vi "DWE Get Time.vi"(9 "Date":string, 10 "# of rows":i32, 11 "Data row":string[][](array[string])) -> (3 "Time array":timestamp[](array[timestamp]))   [LabVIEW 2014]
doc: "Determine and record date of logged data (Laundry.NET does not provide date)."
panel:
  out "Array":bool[](array[boolean])
  out "Numeric":i32
  out "hour":string
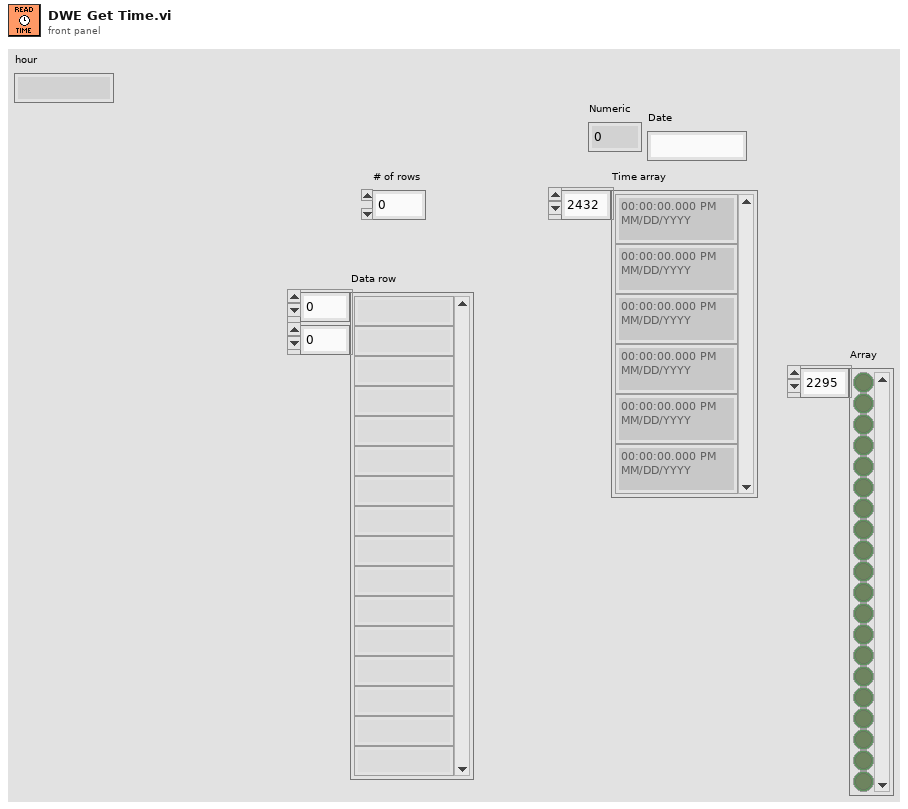
[diagram p1: front panel]
types:
  T1 = typedef "LVDateTimeRec.ctl" = cluster{"fractional second":dbl, "second":i32, "minute":i32, "hour":i32, "day of month":i32, "month":i32, "year":i32, "day of week":i32, "day of year":i32, "DST":i32}
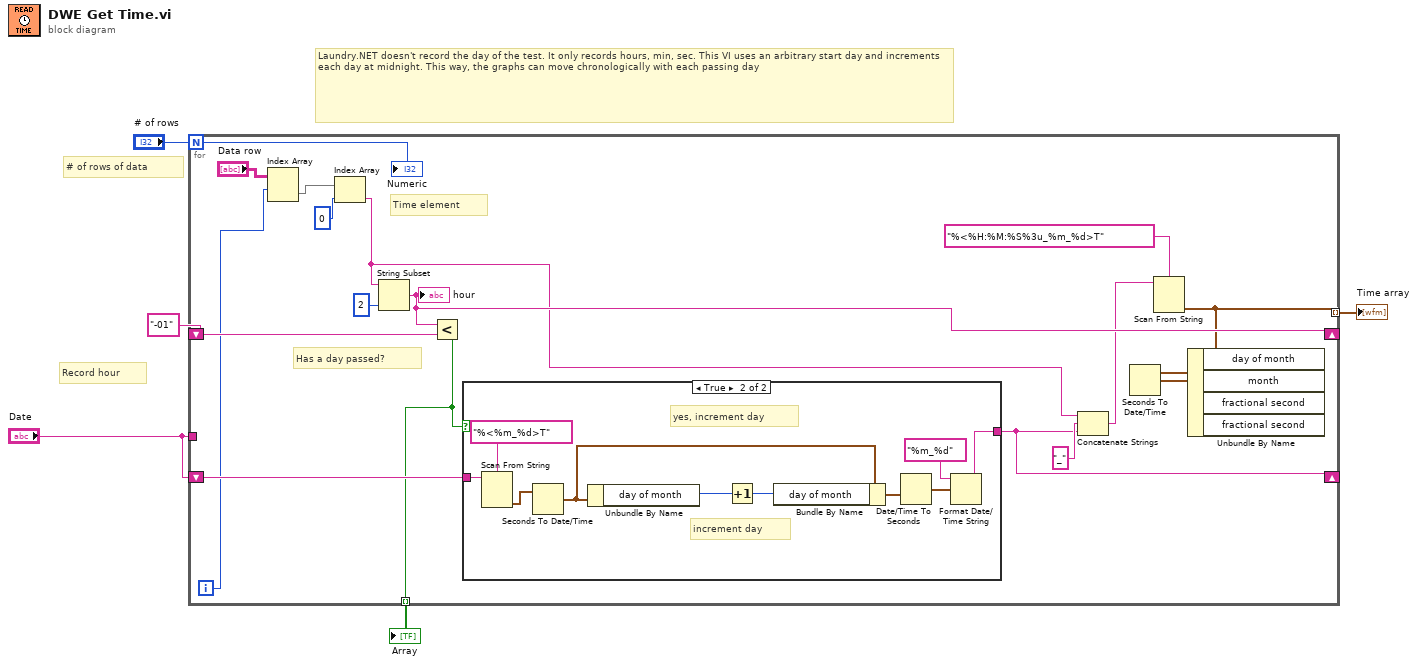
[diagram p0: block diagram]
diagram:
  # "Record hour"
  # "Laundry.NET doesn't record the day of the test. It only records hours, min, sec. This VI uses an arbitrary start day and increments each day at midnight. This way, the graphs can move chronologically with each passing day"
  # "# of rows of data"
  n1 = for {
    N: "# of rows" -> [w13]
    shift-right: [w19] -> _
    shift-left: "-01" ("String") -> [w18]
    tunnel: [w12] -> w4 mode=indexing
    tunnel: "Date" -> [_]
    shift-right: [w8] -> _
    shift-left: "Date" -> [w9]
    tunnel: [w7] -> w1 mode=indexing
    i -> [w6]
    # "Time element"
    # "Has a day passed?"
    n2 = Index Array(array="Data row", index (row)=w6) -> (element=w17:string[])  [unwired: 1 in]
    n3 = Index Array(array=w17, index=0) -> (element=w15:string)
    n4 = String Subset(string=w15, length (rest)=2 ("length (rest)")) -> (substring=w19:string)  [unwired: 1 in]
    "hour" <- w19
    n5 = Less?(x=w19, y=w18) -> (x < y?=w7:bool)
    n6 = case shown="True" w7 {
      tunnel: [w23 w24] -> w8
      tunnel: w9 -> [w23 w25]
      frame False {
        # "No, same day"
      }
      frame True {
        # "increment day"
        # "yes, increment day"
        n7 = Scan From String(format string="%<%m_%d>T", input string=w25) -> (output 1=w32:timestamp)  [unwired: 3 in, 3 out]
        n8 = Seconds To Date/Time(time stamp (now)=w32) -> (date time rec=w30:T1)  [unwired: 1 in]
        n9 = Unbundle By Name(w30) -> ("day of month"=w31:i32)
        n10 = Increment(x=w31) -> (x+1=w29:i32)
        n11 = Bundle By Name(cluster=w30, "day of month"=w29) -> (w28:T1)
        n12 = Date/Time To Seconds(2:w28) -> (0:w27:timestamp)  [unwired: 1 in]
        n13 = Format Date/Time String(time format string (%c)="%m_%d", seconds (now)=w27) -> (date/time string=w24:string)  [unwired: 1 in]
      }
    }
    n14 = Concatenate Strings(w15, "_" ("string"), w8) -> (w14:string)
    n15 = Scan From String(format string="%<%H:%M:%S%3u_%m_%d>T", input string=w14) -> (output 1=w12:timestamp)  [unwired: 3 in, 3 out]
    n16 = Seconds To Date/Time(time stamp (now)=w12) -> (date time rec=w11:T1)  [unwired: 1 in]
    n17 = Unbundle By Name(w11) -> ()  [unwired: 4 out]
    "Numeric" <- w13
  }
  "Time array" <- w4
  "Array" <- w1
